vi "DP-Next Data File.vi"(0 "State in":T1) -> (4 "State out":T1, 6 "run":i32, 8 "data path":path, 15 "error out":errorcluster)   [LabVIEW 2020]
uses:
  CFTS VIs/CFTS-Experiment State.ctl
  epl-vi-lib/Utility VIs/File IO VIs/Configuration File Wrapper VIs/Config-Read Key (string).vi
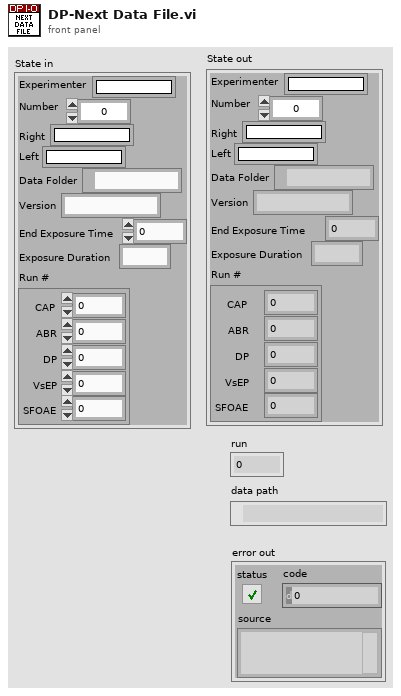
[diagram p1: front panel]
types:
  T1 = typedef "CFTS-Experiment State.ctl" = cluster{"Experimenter":string, "Number":u32, "Right":string, "Left":string, "Data Folder":path, "Version":string, "End Exposure Time":dbl, "Exposure Duration":string, "Run #":cluster{"CAP":i32, "ABR":i32, "DP":i32, "VsEP":i32, "SFOAE":i32}}
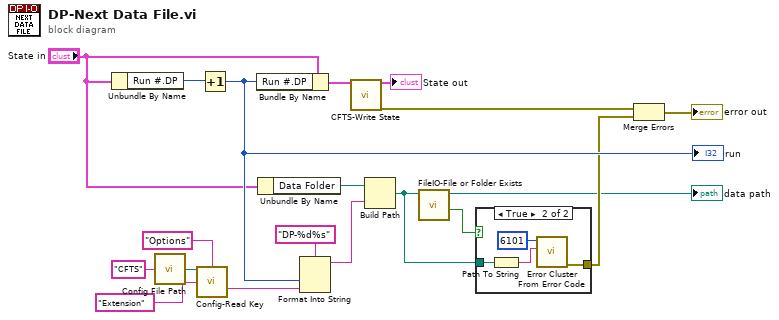
[diagram p0: block diagram]
diagram:
  n1 = Unbundle By Name("State in") -> ("Run #.DP"=w19:i32)
  n2 = call "Config File Path.vi"("AppName"="CFTS") -> ("Default config file name"=w15:path)
  n3 = call-poly "Config-Read Key.vi"("configuration file path"=w15, "section"="Options", "key"="Extension" ("string")) -> ("value"=w11:string)  [unwired: 9 in, 3 out]
  n4 = Increment(x=w19) -> (x+1=w10:i32)
  "run" <- w10
  n5 = Bundle By Name(cluster="State in", "Run #.DP"=w10) -> (w18:T1)
  n6 = Unbundle By Name("State in") -> ("Data Folder"=w9:path)
  n7 = Format Into String(format string="DP-%d%s", w10, w11) -> (resulting string=w6:string)  [unwired: 2 in, 1 out]
  n8 = call "CFTS-Write State.vi"("State"=w18) -> ("State thru"=→"State out":T1, "error out"=w4:errorcluster)  [unwired: 13 in]
  n9 = Build Path(base path=w9, name or relative path=w6) -> (appended path=w7:path)
  n10 = call "FileIO-File or Folder Exists.vi"("path"=w7) -> ("Exists?"=w8:bool, "dup path"=→"data path":path)  [unwired: 7 in, 2 out]
  n11 = case shown="True" w8 {
    tunnel: [_ w23] -> w3
    tunnel: w7 -> [_ w20]
    frame False {
    }
    frame True {
      n12 = Path To String(path=w20) -> (string=w21:string)
      n13 = call <vilib>:"Error Cluster From Error Code.vi"("error message (\"\")"=w21, "error code (0)"=6101) -> ("error out"=w23:errorcluster)  [unwired: 7 in]
    }
  }
  n14 = Merge Errors(w4, w3) -> (→"error out":errorcluster)
